vi "Create Type-Def.vi"() -> ()   [LabVIEW 2018, in "Scripting.lvlib"]
uses:
  Scripting.lvlib
  <vilib>/Utility/sysdir.llb/System Directory Type.ctl
  Event Type-Definition.ctl
panel:
  out "Modifications:VI Modifications Bitset":u64
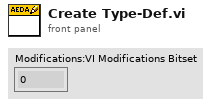
[diagram p1: front panel]
types:
  T1 = enum32{"Invalid", "Standard", "Closed", "Hidden", "Minimized", "Maximized"}
  T2 = enum32{"invalid VI type", "Standard VI", "Control VI", "Global VI", "Polymorphic VI", "Configuration VI", "SubSystem", "Facade VI", "Method VI", "Statechart Diagram VI"}
  T3 = typedef "System Directory Type.ctl" = i32
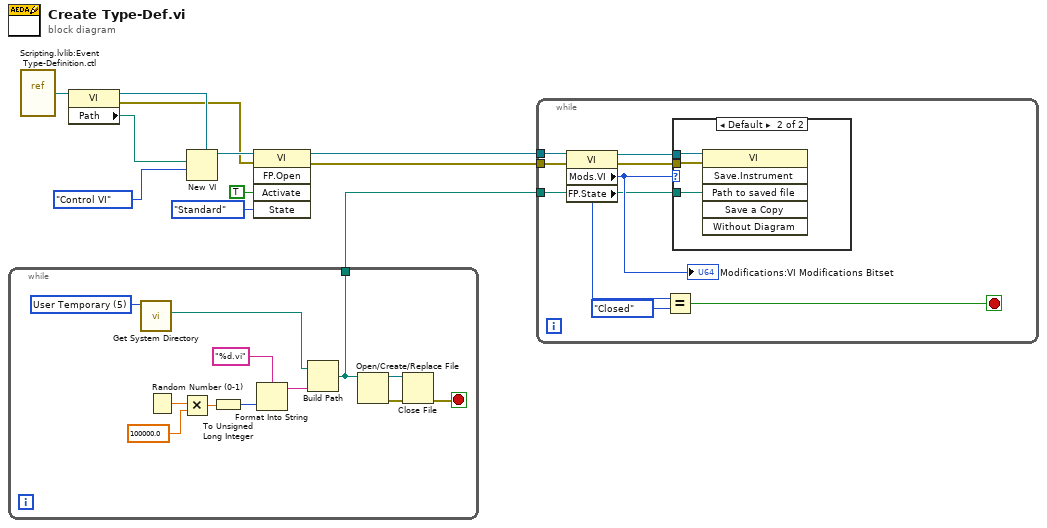
[diagram p0: block diagram]
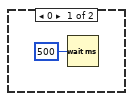
[diagram p2: hidden frame]
diagram:
  n1 = while {
    tunnel: [w12] -> w1
    stop <- w13 stop-if-true
    w23 = T3 5 items=["User Home"=0, "User Desktop"=1, "User Documents"=2, "User Application Data"=3, "User Preferences"=4, "User Temporary"=5, "Public Documents"=6, "Public Application Data"=7, "Public Preferences"=8, "Public Cache"=13, "System Core Libraries"=9, "System Installed Libraries"=10, "Application Files"=11, "Boot Volume Root"=12] ("system directory type")
    n2 = call <vilib>:"Get System Directory.vi"("system directory type"=w23) -> ("system directory"=w22:path)  [unwired: 10 in]
    n3 = Random Number (0-1)() -> (number: 0 to 1=w21:dbl)
    n4 = Multiply(x=w21, y=100000.0) -> (x*y=w19:dbl)
    n5 = To Unsigned Long Integer(number=w19) -> (unsigned 32bit integer=w18:u32)
    n6 = Format Into String(format string="%d.vi", w18) -> (resulting string=w16:string)  [unwired: 2 in, 1 out]
    n7 = Build Path(base path=w22, name or relative path=w16) -> (appended path=w12:path)
    n8 = Open/Create/Replace File(file path (use dialog)=w12) -> (refnum out=w14:refnum<file>, error out=w15:errorcluster)  [unwired: 5 in, 1 out]
    n9 = Close File(refnum=w14, error in=w15) -> (error out=w13:errorcluster)  [unwired: 1 out]
  }
  n10 = vi-ref "Scripting.lvlib:Event Type-Definition.ctl"() -> (w11:refnum<vi>)
  n11 = property class="VI"(reference=w11) -> (reference out=w7:refnum<vi>, error out=w4:errorcluster, "Path"=w10:path)  [unwired: 1 in]
  n12 = New VI(5:w7, 9:T2."Control VI" ("vi type (standard vi)"), 10:w10) -> (3:w8:refnum<vi>)  [unwired: 4 in, 1 out]
  n13 = invoke class="VI" method="FP.Open"(reference=w8, error in=w4, "Activate"=TRUE ("Activate?"), "State"=T1."Standard") -> (reference out=w3:refnum<vi>, error out=w2:errorcluster)  [unwired: 1 in, 3 out]
  n14 = while {
    tunnel: w3 -> [w32]
    tunnel: w2 -> [w31]
    tunnel: w1 -> [w27]
    stop <- w24 stop-if-true
    n15 = property class="VI"(reference=w32, error in=w31) -> (reference out=w29:refnum<vi>, error out=w28:errorcluster, "Mods.VI"=w30:u64, "FP.State"=w26:T1)
    "Modifications:VI Modifications Bitset" <- w30
    n16 = Equal?(x=w26, y=T1."Closed") -> (x = y?=w24:bool)
    n17 = case shown="Default" w30 {
      tunnel: w29 -> [_ w36]
      tunnel: w28 -> [_ w35]
      tunnel: w27 -> [_ w34]
      frame 0 {
        n18 = Wait (ms)(milliseconds to wait=u32 500) -> ()  [unwired: 1 out]
      }
      frame Default {
        n19 = invoke class="VI" method="Save.Instrument"(reference=w36, error in=w35, "Path to saved file"=w34) -> ()  [unwired: 3 in, 6 out]
      }
    }
  }
